vi "Draw List.vi"(8 "error in (no error)":errorcluster, 10 "Highlight Row (-1)":i32=-1, 11 "ScrollingList in":refnum<class "ScrollingList.lvclass">) -> (0 "error out":errorcluster, 3 "ScrollingList out":refnum<class "ScrollingList.lvclass">)   [LabVIEW 2020, in "ScrollingList.lvclass"]
uses:
  ScrollingList.lvclass
  C:/Program Files/National Instruments/LabVIEW 2020/vi.lib/QSI/QControls/QControl Classes/Picture/Picture.lvclass
  C:/Program Files/National Instruments/LabVIEW 2020/vi.lib/QSI/QControls/QControl Classes/GObject/GObject.lvclass
  C:/Program Files/National Instruments/LabVIEW 2020/vi.lib/QSI/QControls/QControl Classes/Control/Control.lvclass
  ScrollingList.lvclass/ScrollingList.ctl
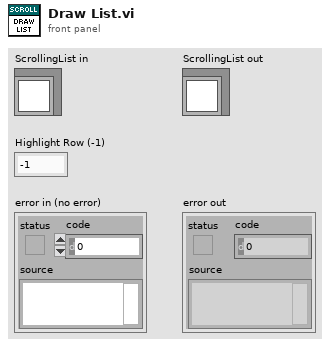
[diagram p1: front panel]
types:
  T1 = cluster{"Font Name:":string, "Size":i16, "Strikeout?":bool, "Italic?":bool, "Underline?":bool, "Outline?":bool, "Shadow?":bool, "Bold?":bool}
  T2 = cluster{"horizontal":enum16{"left", "center", "right"}, "vertical":enum16{"top", "center", "bottom"}}
  T3 = enum16{"User-specified Font", "Application Font", "System Font", "Dialog Font"}
  T4 = typedef "ScrollingList.lvclass/State Data.ctl" = cluster{"Timeout":i32, "Time":timestamp, "Y":i32, "Origin:Top":i16, "Rate":dbl, "ListItems":string[], "Item Height":i32, "Max Height":i32}
  T5 = typedef "LVBoundsTypeDef.ctl" = cluster{"Width":u32, "Height":u32}
  T6 = cluster{"left":i16, "top":i16, "right":i16, "bottom":i16}
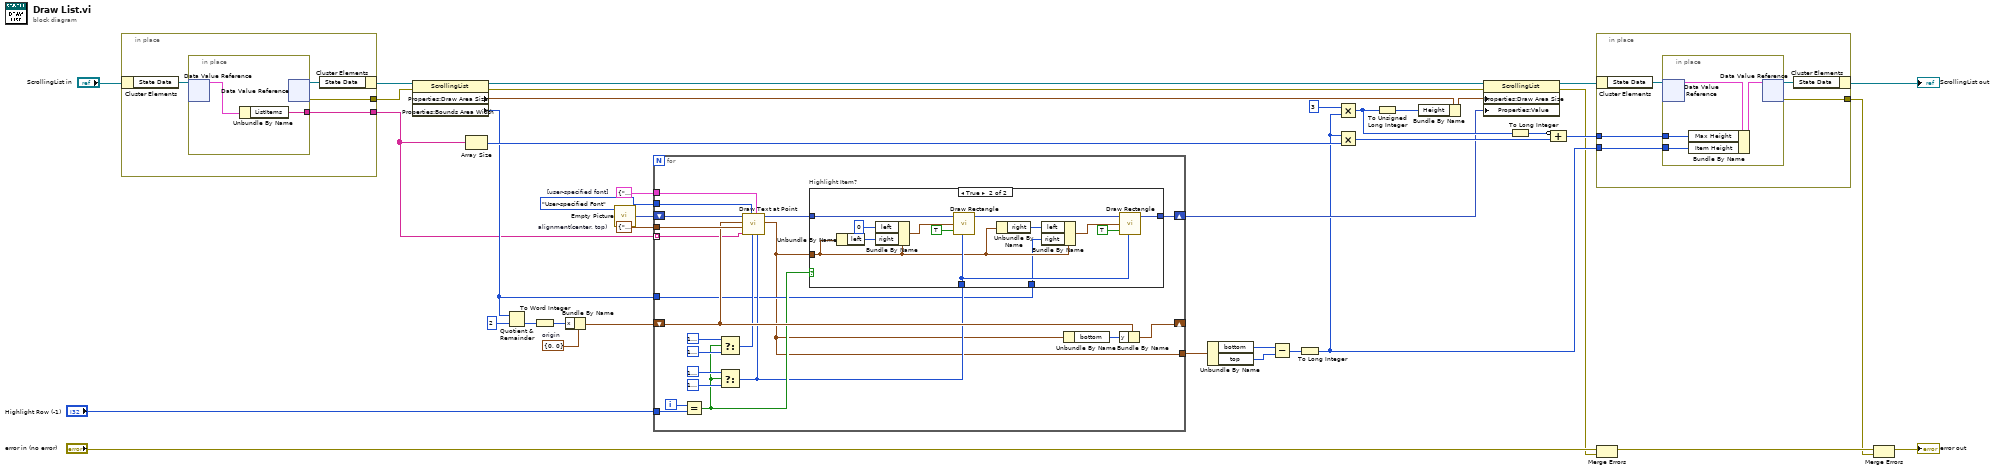
[diagram p0: block diagram]
diagram:
  w26 = T1 {"Font Name:"="Arial", "Size"=60, "Strikeout?"=FALSE, "Italic?"=FALSE, "Underline?"=FALSE, "Outline?"=FALSE, "Shadow?"=FALSE, "Bold?"=FALSE}  # [user-specified font]
  w31 = cluster{"x":i16, "y":i16} {"x"=0, "y"=0}  # origin
  w29 = T2 {"horizontal"=enum."center", "vertical"=enum."top"}  # alignment(center, top)
  n1 = in-place {
    in-place-border: [w42] -> w15
    in-place-border: [w40] -> w37
    n2 = in-place-cluster #1("ScrollingList in") -> ("State Data"=w43:refnum<data-value>)
    n3 = in-place {
      in-place-border: [w44] -> w42
      n4 = in-place-dvr #2(w43) -> (w45:T4)  [unwired: 1 out]
      n5 = Unbundle By Name(w45) -> ("ListItems"=w44:string[])
      n6 = in-place-dvr #2() -> (w41:refnum<data-value>, w40:errorcluster)  [unwired: 1 in]
    }
    n7 = in-place-cluster #1("State Data"=w41) -> (w38:refnum<class "ScrollingList.lvclass">)
  }
  n8 = property on="Property Node" class="ScrollingList"(reference=w38, error in=w37) -> (reference out=w36:refnum<class "ScrollingList.lvclass">, error out=w35:errorcluster, "Properties:Draw Area Size"=w14:T5, "Properties:Bounds Area Width"=w16:u32)
  n9 = Array Size(array=w15) -> (size(s)=w22:i32)
  n10 = Quotient & Remainder(x=w16, y=u32 2) -> (floor(x/y)=w32:u32)  [unwired: 1 out]
  n11 = To Word Integer(number=w32) -> (16bit integer=w30:i16)
  n12 = Bundle By Name(cluster=w31, "x"=w30) -> (w34:cluster{"x":i16, "y":i16})
  n13 = call "Empty Picture"() -> ("empty picture"=w25:picture)
  n14 = for {
    tunnel: T3."User-specified Font" ("desired font(Application)") -> [w64]
    tunnel: w26 -> [w63]
    tunnel: w29 -> [w62]
    shift-right: [w47] -> w12
    shift-left: w25 -> [w60]
    shift-right: [w65] -> _
    shift-left: w34 -> [w61]
    tunnel: w15 -> [w59] mode=indexing
    tunnel: [w46] -> w24
    tunnel: "Highlight Row (-1)" -> [w57]
    tunnel: w16 -> [w48]
    i -> [w58]
    n15 = Equal?(x=w58, y=w57) -> (x = y?=w50:bool)
    n16 = Select(t=u32 16777225, s=w50, f=u32 16777222) -> (s? t:f=w54:u32)
    n17 = Select(t=u32 16777224, s=w50, f=u32 16777216) -> (s? t:f=w49:u32)
    n18 = call <vilib>:"Draw Text at Point.vi"("BG color(transparent)"=w49, "[user-specified font]"=w63, "text color(black)"=w54, "desired font(Application)"=w64, "text"=w59, "alignment(left, top)"=w62, "origin"=w61, "picture"=w60) -> ("text rect"=w46:T6, "new picture"=w51:picture)  [unwired: 2 in]
    n19 = case "Highlight Item?" shown="True" w50 {
      tunnel: w51 -> [w67 w80]
      tunnel: w49 -> [_ w76]
      tunnel: w46 -> [_ w70]
      tunnel: w48 -> [_ w68]
      tunnel: [w67 w75] -> w47
      frame False {
      }
      frame True {
        n20 = Unbundle By Name(w70) -> ("left"=w74:i16)
        n21 = Bundle By Name(cluster=w70, "left"=i16 0, "right"=w74) -> (w72:T6)
        n22 = call <vilib>:"Draw Rectangle.vi"("picture"=w80, "rect"=w72, "fill?(F)"=TRUE, "color(black)"=w76) -> ("new picture"=w78:picture)  [unwired: 5 in]
        n23 = Unbundle By Name(w70) -> ("right"=w69:i16)
        n24 = Bundle By Name(cluster=w70, "left"=w69, "right"=w68) -> (w71:T6)
        n25 = call <vilib>:"Draw Rectangle.vi"("picture"=w78, "rect"=w71, "fill?(F)"=TRUE, "color(black)"=w76) -> ("new picture"=w75:picture)  [unwired: 5 in]
      }
    }
    n26 = Unbundle By Name(w46) -> ("bottom"=w66:i16)
    n27 = Bundle By Name(cluster=w61, "y"=w66) -> (w65:cluster{"x":i16, "y":i16})
  }
  n28 = Unbundle By Name(w24) -> ("bottom"=w28:i16, "top"=w23:i16)
  n29 = Subtract(x=w28, y=w23) -> (x-y=w19:i16)
  n30 = To Long Integer(number=w19) -> (32bit integer=w9:i32)
  n31 = Multiply(x=3 ("y"), y=w9) -> (x*y=w18:i32)
  n32 = Multiply(x=w9, y=w22) -> (x*y=w21:i32)
  n33 = To Unsigned Long Integer(number=w18) -> (unsigned 32bit integer=w6:u32)
  n34 = Bundle By Name(cluster=w14, "Height"=w6) -> (w13:T5)
  n35 = property on="Property Node" class="ScrollingList"(reference=w36, error in=w35, "Properties:Draw Area Size"=w13, "Properties:Value"=w12) -> (reference out=w11:refnum<class "ScrollingList.lvclass">, error out=w4:errorcluster)
  n36 = To Long Integer(number=w18) -> (32bit integer=w20:i32)
  n37 = Compound Arithmetic op=ADD(invert w20, w21) -> (w8:i32)
  n38 = in-place {
    in-place-border: [w83] -> w2
    in-place-border: w9 -> [w82]
    in-place-border: w8 -> [w81]
    n39 = in-place-cluster #3(w11) -> ("State Data"=w85:refnum<data-value>)
    n40 = in-place {
      in-place-border: w82 -> [w88]
      in-place-border: w81 -> [w86]
      n41 = in-place-dvr #4(w85) -> (w89:T4)  [unwired: 1 out]
      n42 = Bundle By Name(cluster=w89, "Max Height"=w86, "Item Height"=w88) -> (w87:T4)
      n43 = in-place-dvr #4(w87) -> (w84:refnum<data-value>, w83:errorcluster)
    }
    n44 = in-place-cluster #3("State Data"=w84) -> (→"ScrollingList out":refnum<class "ScrollingList.lvclass">)
  }
  n45 = Merge Errors("error in (no error)", w4) -> (w5:errorcluster)
  n46 = Merge Errors(w5, w2) -> (→"error out":errorcluster)
